vi "OptoOnStateMachine_2016_5_31_1654.vi"(6 "Touch 1":bool, 7 "State Machine States":T1(ring), 9 "Opto On Time 1 (mSec)":u32=5000, 10 "Tick Count(uSec) in":u32, 11 "TurnOnOpto 1":bool) -> (1 "Boolean":bool, 2 "State Machine States OUT":T1(ring), 3 "Tick Count(uSec) out":u32, 4 "Start Tick Count":u32, 5 "ON Duration (usec)":u32)   [LabVIEW 2013]
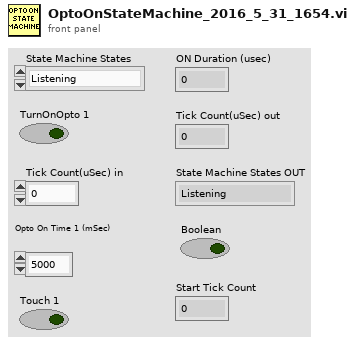
[diagram p1: front panel]
types:
  T1 = enum16{"Listening", "Turn ON", "Timing", "Turn OFF"}
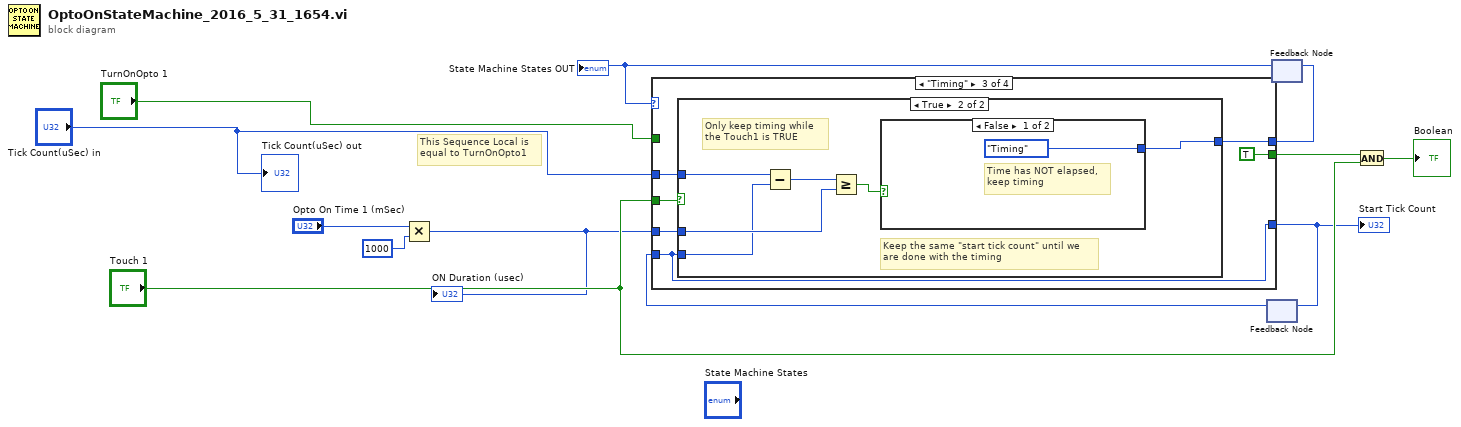
[diagram p0: block diagram]
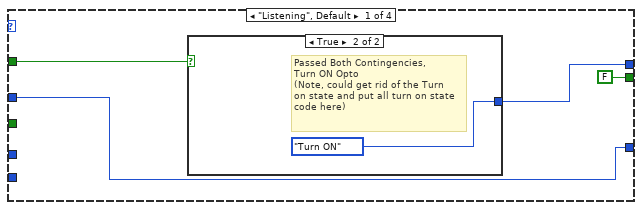
[diagram p2: hidden frame]
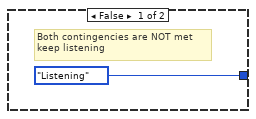
[diagram p3: hidden frame]
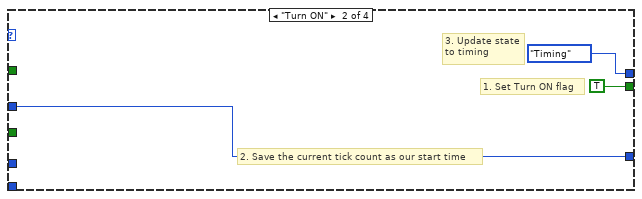
[diagram p4: hidden frame]
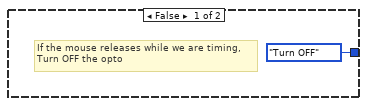
[diagram p5: hidden frame]
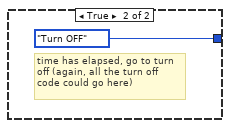
[diagram p6: hidden frame]
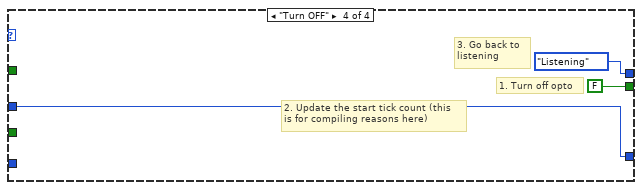
[diagram p7: hidden frame]
diagram:
  # "This Sequence Local is\nequal to TurnOnOpto1"
  n1 = Multiply(x="Opto On Time 1 (mSec)", y=u32 1000) -> (x*y=w7:u32)
  "ON Duration (usec)" <- w7
  n2 = feedback #1() -> (w5:u32)  [unwired: 1 in]
  n3 = feedback #2() -> (w3:T1)  [unwired: 1 in]
  "State Machine States OUT" <- w3
  n4 = case shown="\"Timing\"" w3 {
    tunnel: "TurnOnOpto 1" -> [w16 _ _ _]
    tunnel: w7 -> [_ _ w27 _]
    tunnel: "Tick Count(uSec) in" -> [w14 w21 w24 w39]
    tunnel: [w15 T1."Timing" ("State Machine States") w26 T1."Listening" ("State Machine States")] -> w2
    tunnel: [w14 w21 w23 w39] -> w4
    tunnel: w5 -> [_ _ w23 _]
    tunnel: [FALSE ("Opto on 1") TRUE ("Opto on 1") TRUE ("Opto on 1") FALSE ("Opto on 1")] -> w10
    tunnel: "Touch 1" -> [_ _ w22 _]
    frame "Listening", Default {
      n5 = case shown="True" w16 {
        tunnel: [T1."Listening" ("State Machine States") T1."Turn ON" ("State Machine States")] -> w15
        frame False {
          # "Both contingencies are NOT met\nkeep listening"
        }
        frame True {
          # "Passed Both Contingencies, \nTurn ON Opto\n(Note, could get rid of the Turn\non state and put all turn on state\ncode here)"
        }
      }
    }
    frame "Turn ON" {
      # "3. Update state\nto timing"
      # "2. Save the current tick count as our start time"
      # "1. Set Turn ON flag"
    }
    frame "Timing" {
      n6 = case shown="True" w22 {
        tunnel: w27 -> [_ w33]
        tunnel: [T1."Turn OFF" ("State Machine States") w31] -> w26
        tunnel: w24 -> [_ w30]
        tunnel: w23 -> [_ w29]
        frame False {
          # "If the mouse releases while we are timing,\nTurn OFF the opto"
        }
        frame True {
          # "Only keep timing while\nthe Touch1 is TRUE"
          # "Keep the same \"start tick count\" until we\nare done with the timing"
          n7 = Subtract(x=w30, y=w29) -> (x-y=w34:u32)
          n8 = Greater Or Equal?(x=w34, y=w33) -> (x >= y?=w32:bool)
          n9 = case shown="False" w32 {
            tunnel: [T1."Timing" ("State Machine States") T1."Turn OFF" ("State Machine States")] -> w31
            frame False {
              # "Time has NOT elapsed,\nkeep timing"
            }
            frame True {
              # "time has elapsed, go to turn\noff (again, all the turn off\ncode could go here)"
            }
          }
        }
      }
    }
    frame "Turn OFF" {
      # "2. Update the start tick count (this \nis for compiling reasons here)"
      # "3. Go back to \nlistening"
      # "1. Turn off opto"
    }
  }
  "Start Tick Count" <- w4
  n10 = feedback-in #1(w4) -> ()
  n11 = feedback-in #2(w2) -> ()
  n12 = And(x=w10, y="Touch 1") -> (x .and. y?=→"Boolean":bool)
  "Tick Count(uSec) out" <- "Tick Count(uSec) in"
